vi "水样测试配置.vi"() -> (2 "确认输出":bool, 3 "水样测定时间输出":dbl=1.0)   [LabVIEW 2016, in "国弘多参数.lvlib"]
uses:
  <vilib>/Utility/config.llb/NI_LVConfig.lvlib
panel:
  in  "取消":bool
  in  "确定":bool
  in  "水样测试时间":dbl=1.0
  # "请输入水样测定时间"
  # "min"
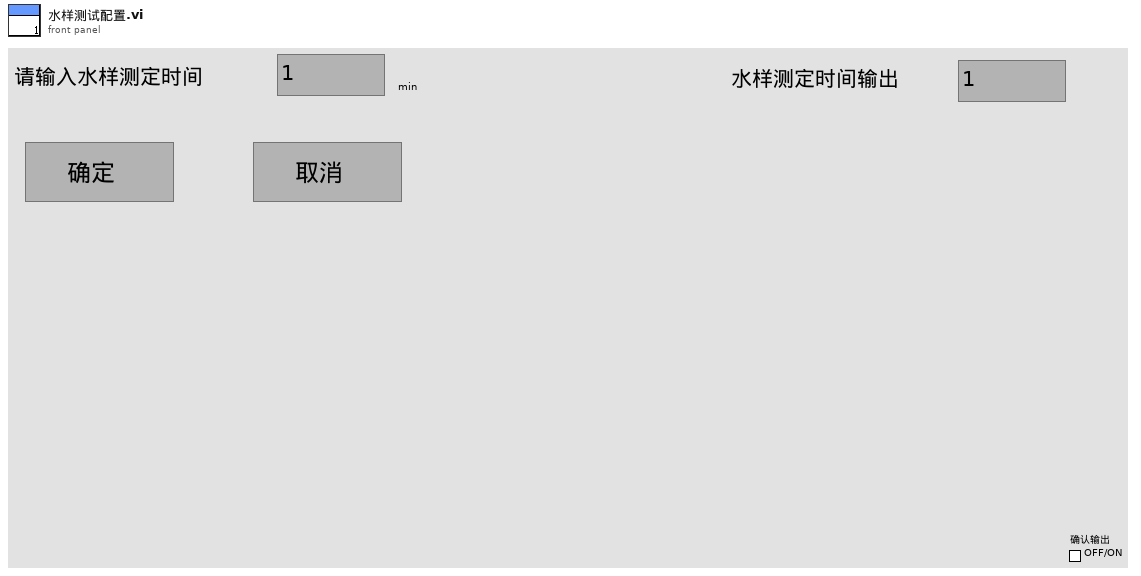
[diagram p1: front panel]
types:
  T1 = typedef "NI_LVConfig.lvlib/Config Data RefNum.ctl" = refnum<k1>
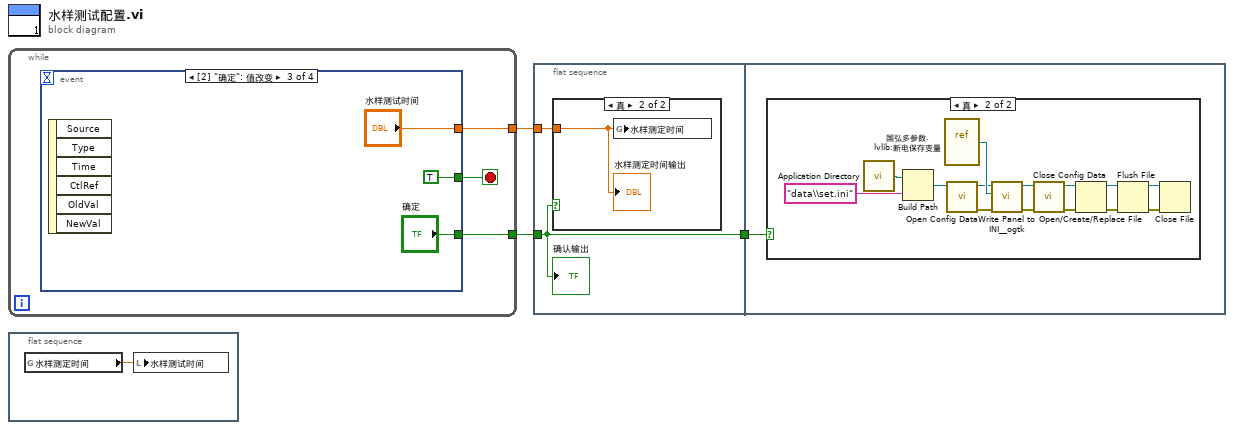
[diagram p0: block diagram]
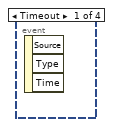
[diagram p4: hidden frame]
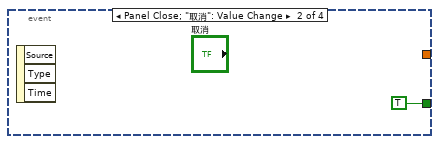
[diagram p5: hidden frame]
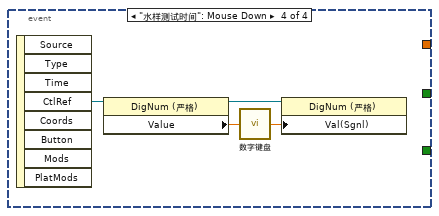
[diagram p6: hidden frame]
diagram:
  n1 = while {
    tunnel: [w5] -> w2
    tunnel: [w4] -> w3
    stop <- w6 stop-if-true
    n2 = event shown="[2] \"确定\": 值改变" {
      selector: _ -> [_ _ _ _]
      dyn-events: _ -> [_ _ _ _]
      timeout: _ -> [_ _ _ _]
      tunnel: [_ TRUE TRUE _] -> w6
      tunnel: [_ _ "水样测试时间" _] -> w5
      tunnel: [_ _ "确定" _] -> w4
      event Timeout {
        n3 = event-data() -> ()  [unwired: 1 in, 3 out]
      }
      event Panel Close; "取消": Value Change {
        n4 = event-data() -> ()  [unwired: 1 in, 3 out]
      }
      event "确定": Value Change {
        n5 = event-data() -> ()  [unwired: 1 in, 6 out]
      }
      event "水样测试时间": Mouse Down {
        n6 = event-data() -> ("CtlRef"=w14:refnum<vi>)  [unwired: 1 in, 7 out]
        n7 = property class="DigNum (严格)"(reference=w14) -> (reference out=w11:refnum<vi>, "Value"=w13:dbl)  [unwired: 1 in, 1 out]
        n8 = call "数字键盘.vi"("OldNumber"=w13) -> ("NewNumber"=w12:sgl)
        n9 = property class="DigNum (严格)"(reference=w11, "Val(Sgnl)"=w12) -> ()  [unwired: 1 in, 2 out]
      }
    }
  }
  n10 = flat-sequence {
    frame #0 {
      n11 = global read "断电保存变量.vi" "水样测定时间"() -> (w15:dbl)
      n12 = local write "水样测试时间"(w15) -> ()
    }
  }
  n13 = flat-sequence {
    tunnel: w3 -> [w16]
    tunnel: w2 -> [w17]
    tunnel: [w16] -> w1
    tunnel: w1 -> [w19]
    frame #0 {
      n14 = case shown="真" w16 {
        tunnel: w17 -> [_ w18]
        frame False {
        }
        frame True {
          n15 = global write "断电保存变量.vi" "水样测定时间"(w18) -> ()
          "水样测定时间输出" <- w18
        }
      }
      "确认输出" <- w16
    }
    frame #1 {
      n16 = case shown="真" w19 {
        frame False {
        }
        frame True {
          n17 = call <vilib>:"Application Directory.vi"() -> ("Application Directory"=w24:path)
          n18 = Build Path(base path=w24, name or relative path="data\\set.ini" ("名称或相对路径")) -> (appended path=w25:path)
          n19 = vi-ref "国弘多参数.lvlib:断电保存变量.vi"() -> (w27:refnum<vi>)
          n20 = call <vilib>:"Open Config Data.vi"("configuration file path"=w25) -> ("error out"=w21:errorcluster, "refnum"=w20:T1)  [unwired: 8 in, 1 out]
          n21 = call <userlib>:"Write Panel to INI__ogtk.vi"("error in (no error)"=w21, "VI ref"=w27, "refnum"=w20) -> ("error out"=w23:errorcluster, "refnum out"=w22:T1)  [unwired: 7 in]
          n22 = call <vilib>:"Close Config Data.vi"("error in (no error)"=w23, "refnum"=w22) -> ("error out"=w31:errorcluster, "file path"=w30:path)  [unwired: 8 in]
          n23 = Open/Create/Replace File(file path (use dialog)=w30, error in=w31) -> (refnum out=w29:refnum<file>, error out=w28:errorcluster)  [unwired: 4 in, 1 out]
          n24 = Flush File(refnum=w29, error in=w28) -> (refnum out=w33:refnum<file>, error out=w32:errorcluster)
          n25 = Close File(refnum=w33, error in=w32) -> ()  [unwired: 2 out]
        }
      }
    }
  }
